vi "Coil V to Temp.vi"(2 "Coil Specs":T1 {"Coil Coefficients" format="%.3e"; "Temp Coef" format="%.5f"}, 3 "T inlet":dbl format="%.2f", 4 "I":dbl format="%.2f", 5 "V":dbl[](array[numeric]) format="%.2f") -> (0 "I*Coil Temperature":dbl[](array[numeric]) format="%.2f", 1 "Expected Voltage":dbl[](array[numeric]) format="%.2f")   [LabVIEW 2019]
doc: "Calculates the expected voltage from the inlet water temperature, coil currents and coil resistance coefficients. Also calculates the product of the current and the average coil temperature from the coil voltages, coil currents and the zero current coil resistance. Assumes a temperature coefficient for Cu of 4e-3.\nScott Hannahs, NHMFL-FSU, April 1995"
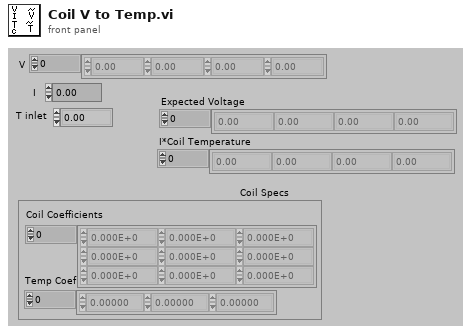
[diagram p1: front panel]
types:
  T1 = cluster{"Coil Coefficients":dbl[][], "Temp Coef":dbl[]}
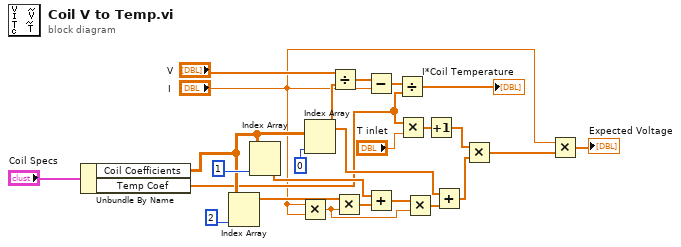
[diagram p0: block diagram]
diagram:
  n1 = Unbundle By Name("Coil Specs") -> ("Coil Coefficients"=w4:dbl[][], "Temp Coef"=w3:dbl[])
  n2 = Index Array(array=w4, index (col)=2) -> (element=w11:dbl[])  [unwired: 1 in]
  n3 = Index Array(array=w4, index (col)=1) -> (element=w12:dbl[])  [unwired: 1 in]
  n4 = Multiply(x="I", y="I") -> (x*y=w7:dbl)
  n5 = Index Array(array=w4, index (col)=0) -> (element=w13:dbl[])  [unwired: 1 in]
  n6 = Divide(x="V", y=w13) -> (x/y=w24:dbl[])
  n7 = Multiply(x=w11, y=w7) -> (x*y=w16:dbl[])
  n8 = Subtract(x=w24, y="I") -> (x-y=w6:dbl[])
  n9 = Add(x=w12, y=w16) -> (x+y=w15:dbl[])
  n10 = Divide(x=w6, y=w3) -> (x/y=→"I*Coil Temperature":dbl[])
  n11 = Multiply(x=w3, y="T inlet") -> (x*y=w21:dbl[])
  n12 = Multiply(x=w15, y=w7) -> (x*y=w17:dbl[])
  n13 = Increment(x=w21) -> (x+1=w20:dbl[])
  n14 = Add(x=w13, y=w17) -> (x+y=w14:dbl[])
  n15 = Multiply(x=w20, y=w14) -> (x*y=w18:dbl[])
  n16 = Multiply(x="I", y=w18) -> (x*y=→"Expected Voltage":dbl[])
